vi "Archive Directories.vi"(8 "Error In":errorcluster, 9 "Archive Dest":path=path "C:/Program Files/National Instruments/LabVIEW 2013/vi.lib/LabVIEW Hacker/EZ430-Chronos-Interface-bak.zip", 10 "Archive Root":path=path "C:/Program Files/National Instruments/LabVIEW 2013", 11 "Directory Paths":path[](array[path])=[path "C:/Program Files/National Instruments/LabVIEW 2013/vi.lib/LabVIEW Hacker/EZ430-Chronos-Interface", path "C:/Program Files/National Instruments/LabVIEW 2013/examples/LabVIEW Hacker/EZ430-Chronos-Interface", path "C:/Program Files/National Instruments/LabVIEW 2013/examples/exbins/LabVIEW Hacker/EZ430-Chronos-Interface", path "C:/Program Files/National Instruments/LabVIEW 2013/menus/Categories/EZ430-Chronos"]) -> (0 "Error Out":errorcluster)   [LabVIEW 2011, in "LVH-Toolbox.lvlib" / "LVH-SystemTools.lvlib"]
doc: "Build archive containing multiple folders. Archive Root is a parent folder common to all Directory Paths. All files are stored in the archive relative to archive root."
uses:
  LVH-SystemTools.lvlib
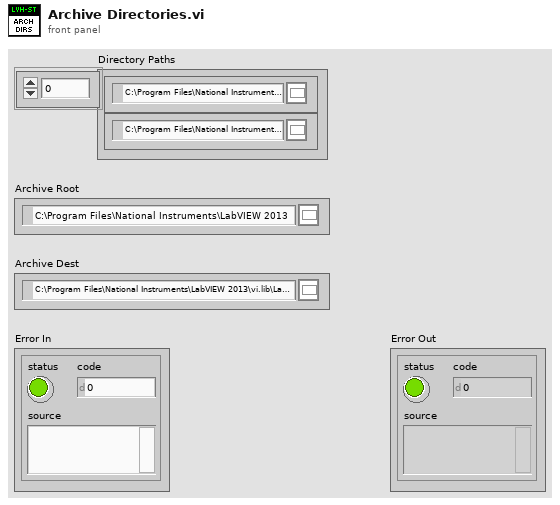
[diagram p1: front panel]
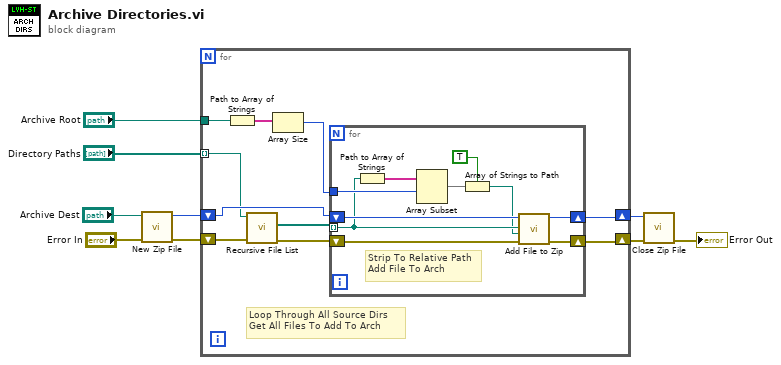
[diagram p0: block diagram]
diagram:
  n1 = call <vilib>:"New Zip File.vi"("error in (no error)"="Error In", "target"="Archive Dest") -> ("error out"=w3:errorcluster, "zip file out"=w8:i64)  [unwired: 3 in, 1 out]
  n2 = for {
    tunnel: "Directory Paths" -> [w11] mode=indexing
    shift-right: [w17] -> w7
    shift-left: w3 -> [w13]
    shift-right: [w16] -> w6
    shift-left: w8 -> [w18]
    tunnel: "Archive Root" -> [w10]
    # "Loop Through All Source Dirs\nGet All Files To Add To Arch"
    n3 = Path to Array of Strings(0:w10) -> (2:w15:string[])  [unwired: 1 out]
    n4 = call <vilib>:"Recursive File List.vi"("error in (no error)"=w13, "Folder Path"=w11) -> ("error out"=w12:errorcluster, "All Files in Dir"=w19:path[])  [unwired: 5 in, 3 out]
    n5 = Array Size(array=w15) -> (size(s)=w14:i32)
    n6 = for {
      tunnel: w19 -> [w21] mode=indexing
      shift-right: [w26] -> w17
      shift-left: w12 -> [w28]
      shift-right: [w27] -> w16
      shift-left: w18 -> [w29]
      tunnel: w14 -> [w22]
      # "Strip To Relative Path\nAdd File To Arch"
      n7 = Path to Array of Strings(0:w21) -> (2:w25:string[])  [unwired: 1 out]
      n8 = Array Subset(array=w25, index=w22) -> (w24:string[])  [unwired: 1 in]
      n9 = Array of Strings to Path(0:w24, 1:TRUE ("relative")) -> (2:w20:path)
      n10 = call <vilib>:"Add File to Zip.vi"("error in (no error)"=w28, "destination path in zip"=w20, "source file path"=w21, "zip file in"=w29) -> ("error out"=w26:errorcluster, "zip file out"=w27:i64)  [unwired: 6 in]
    }
  }
  n11 = call <vilib>:"Close Zip File.vi"("error in (no error)"=w7, "zip file in"=w6) -> ("error out"=→"Error Out":errorcluster)  [unwired: 5 in]
